vi "Module Type.vi"(11 "ValveSimModule in":refnum<class "ValveSimModule.lvclass">) -> (2 "Module Type":string)   [LabVIEW 2020, in "VolatusScratch.lvlib" / "ValveSimModule.lvclass"]
uses:
  ValveSimModule.lvclass
  ValveSimModule.lvclass/ValveSimModule.ctl
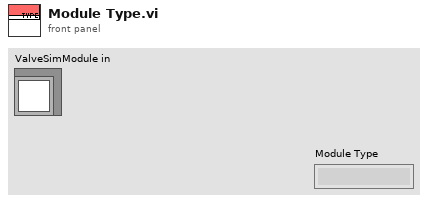
[diagram p1: front panel]
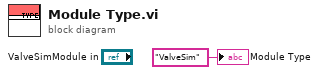
[diagram p0: block diagram]
diagram:
  "Module Type" <- "ValveSim" ("Module Type")
